vi "XML Single Element Attribute String.vi"(9 "prop-val pairs":string[][](array[string]), 10 "name":string, 11 "Base":string) -> (3 "Attribute string":string)   [LabVIEW 2012]
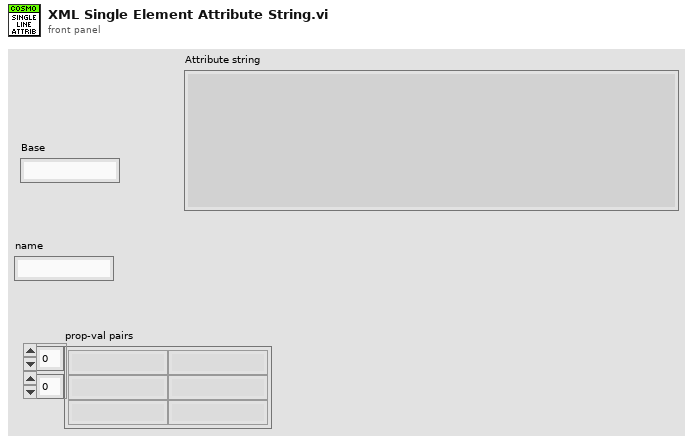
[diagram p1: front panel]
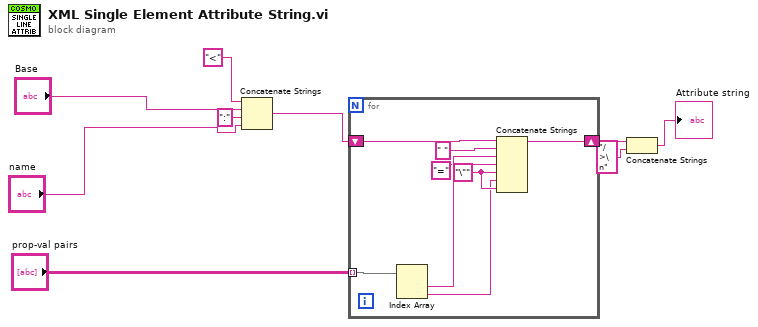
[diagram p0: block diagram]
diagram:
  n1 = Concatenate Strings("<" ("string"), "Base", ":" ("string"), "name") -> (w5:string)
  n2 = for {
    shift-right: [w12] -> w3
    shift-left: w5 -> [w16]
    tunnel: "prop-val pairs" -> [w17] mode=indexing
    w11 = "\"" ("string")
    n3 = Index Array(array=w17) -> (element #1=w14:string, element #2=w10:string)  [unwired: 2 in]
    n4 = Concatenate Strings(w16, " " ("string"), w14, "=" ("string"), w11, w10, w11) -> (w12:string)
  }
  n5 = Concatenate Strings(w3, "/>\n" ("string")) -> (→"Attribute string":string)
